vi "set_remote_lock_enable_status.vi"(8 "error in (no error)":errorcluster, 10 "Enable":bool, 11 "VISA resource name":refnum<visa-resource-name>) -> (0 "error out":errorcluster, 3 "VISA resource name out":refnum<visa-resource-name>)   [LabVIEW 2018]
doc: "Enable or disable the remote lock.\n\nWhen the remote lock is enabled, no parameters can be updated from the instrument front panel. \"R Lock\" will be displayed on the instrument."
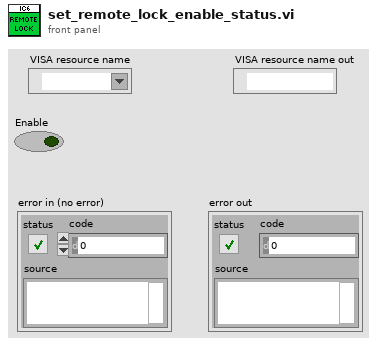
[diagram p1: front panel]
types:
  T1 = enum16{"Source", "General", "Input name", "Process name", "Logic", "Material", "Material name", "Output name", "Process", "Sensor", "Output type", "User message", "Layer", ""}
  T2 = enum16{"Hello", "Query", "Remote action", "Status", "Update"}
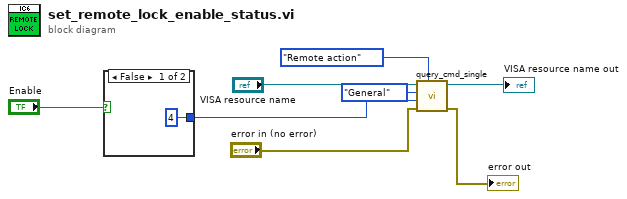
[diagram p0: block diagram]
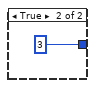
[diagram p2: hidden frame]
diagram:
  n1 = case shown="False" "Enable" {
    tunnel: [u8 4 ("Command ID") u8 3 ("Command ID")] -> w5
    frame False {
    }
    frame True {
    }
  }
  n2 = call "query_cmd_single.vi"("Command group"=T2."Remote action", "error in (no error)"="error in (no error)", "Command ID"=w5, "Command subgroup"=T1."General", "VISA resource name"="VISA resource name") -> ("error out"=→"error out":errorcluster, "VISA resource name out"=→"VISA resource name out":refnum<visa-resource-name>)  [unwired: 2 in, 3 out]
